vi "DSF.Engine.Interface.Read.Error.vi"(8 "error in (no error)":errorcluster, 9 "timeout in ms (0)":i32, 11 "Interface in":refnum<class "DSF.Engine.Interface.lvclass">) -> (0 "error out":errorcluster, 1 "timed out?":bool, 2 "error":errorcluster, 3 "Interface out":refnum<class "DSF.Engine.Interface.lvclass">)   [LabVIEW 2017, in "DSF.Engine.lvlib" / "DSF.Engine.Interface.lvclass"]
uses:
  DSF.Engine.Interface.lvclass
  DSF.Engine.Interface.lvclass/DSF.Engine.Interface.ctl
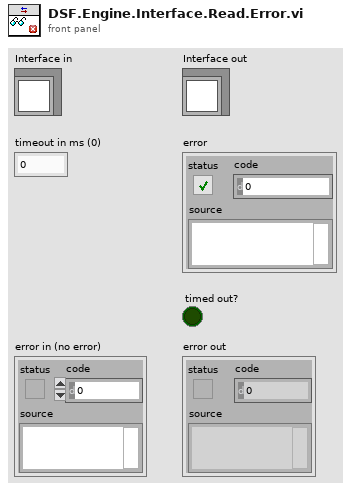
[diagram p1: front panel]
types:
  T1 = typedef "DSF.Engine.lvlib/DSF.Engine.Interface.lvclass/DSF.Engine.Interface.Error Queue.Ref.ctl" = refnum<queue>
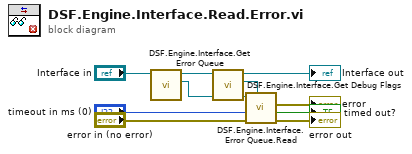
[diagram p0: block diagram]
diagram:
  n1 = call "DSF.Engine.Interface.Get Error Queue.vi"("Interface in"="Interface in") -> ("Error Queue"=w10:T1, "Interface out"=w6:refnum<class "DSF.Engine.Interface.lvclass">)  [unwired: 9 in]
  n2 = call "DSF.Engine.Interface.Get Debug Flags.vi"("Interface in"=w6) -> ("FIFO Debug Flags"=w5:refnum<class "DSF.Engine.Debug Flags.FIFO.lvclass">, "Interface out"=→"Interface out":refnum<class "DSF.Engine.Interface.lvclass">)  [unwired: 9 in]
  n3 = call "DSF.Engine.Interface.Error Queue.Read.vi"("FIFO Debug Flags"=w5, "error in (no error)"="error in (no error)", "timeout in ms (0)"="timeout in ms (0)", "Error Queue in"=w10) -> ("error out"=→"error out":errorcluster, "timed out?"=→"timed out?":bool, "element"=→"error":errorcluster)  [unwired: 4 in, 1 out]
